vi "Get Acquired Data.vi"(8 "error in (no error)":errorcluster, 11 "CCDCamera in":refnum<class "CCDCamera.lvclass">) -> (0 "error out":errorcluster, 3 "CCDCamera out":refnum<class "CCDCamera.lvclass">)   [LabVIEW 2018, in "CCDCamera.lvclass"]
doc: "Este VI faz a leitura da última imagem obtida pela CCD."
uses:
  CCDCamera.lvclass
  CCDCamera.lvclass/CCDCamera.ctl
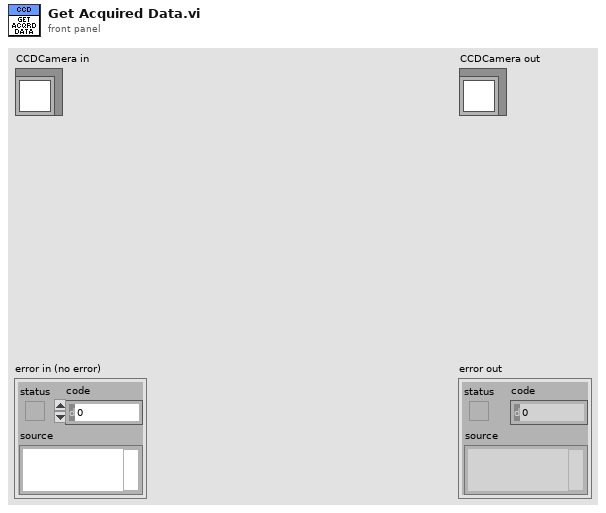
[diagram p1: front panel]
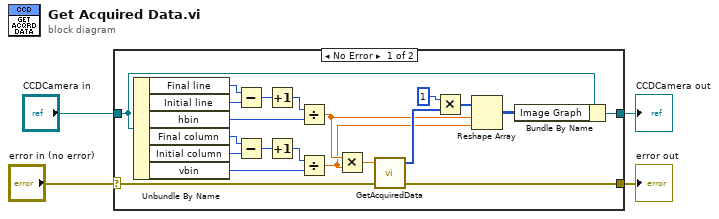
[diagram p0: block diagram]
diagram:
  n1 = case shown="No Error" "error in (no error)" {
    selector: "error in (no error)" -> [w22 w27]
    tunnel: [w21 w27] -> w3
    tunnel: [w19 w26] -> w1
    tunnel: "CCDCamera in" -> [w20 w26]
    frame No Error {
      n2 = Unbundle By Name(w20) -> ("Final line"=w16:u32, "Initial line"=w15:u16, "hbin"=w9:u16, "Final column"=w14:u32, "Initial column"=w13:u16, "vbin"=w6:u16)
      n3 = Subtract(x=w16, y=w15) -> (x-y=w12:u32)
      n4 = Subtract(x=w14, y=w13) -> (x-y=w11:u32)
      n5 = Increment(x=w12) -> (x+1=w10:u32)
      n6 = Increment(x=w11) -> (x+1=w7:u32)
      n7 = Divide(x=w10, y=w9) -> (x/y=w8:dbl)
      n8 = Divide(x=w7, y=w6) -> (x/y=w5:dbl)
      n9 = Multiply(x=w8, y=w5) -> (x*y=w18:dbl)
      n10 = call <userlib>:"GetAcquiredData.vi"("error in (no error)"=w22, "size"=w18) -> ("error out"=w21:errorcluster, "array"=w24:i32[])  [unwired: 1 in, 1 out]
      n11 = Multiply(x=1, y=w24) -> (x*y=w25:i32[])
      n12 = Reshape Array(w25, w8, w5) -> (w17:i32[][])
      n13 = Bundle By Name(cluster=w20, "Image Graph"=w17) -> (w19:refnum<class "CCDCamera.lvclass">)
    }
    frame Error {
    }
  }
  "error out" <- w3
  "CCDCamera out" <- w1
